vi "Update Occupied Area.vi"(8 "error in (no error)":errorcluster, 11 "UI Controller in":refnum<class "UI Controller.lvclass">) -> (0 "error out":errorcluster, 3 "UI Controller out":refnum<class "UI Controller.lvclass">)   [LabVIEW 2015, in "UI Controller.lvlib" / "UI Controller.lvclass"]
uses:
  UI Controller.lvclass
  UI Controller.lvclass/UI Controller.ctl
  <vilib>/ActorFrameworkMVC/View Controller/View Controller/View Controller.lvclass
panel:
  # "NOTICE -- YOU MUST LEAVE THIS NOTICE IN PLACE.\n\nCopyright (c) 2015, LIANG LIU Shawn.Liu.cn@gmail.com\nAll rights reserved.\n\nRedistribution and use in source and binary forms, with or without modification, are permitted provided that the following conditions are met:\n-Redistributions of source code must retain the above copyright notice, this list of conditions and the following disclaimer.\n-Redistributions in binary form must reproduce the above copyright notice, this list of conditions and the following disclaimer in the documentation and/or other materials provided with the distribution.\n-Neither the name of the eLp nor the names of its contributors may be used to endorse or promote products derived from this software without specific prior written permission.\n\nTHIS SOFTWARE IS PROVIDED BY THE COPYRIGHT HOLDERS AND CONTRIBUTORS \"AS IS\" AND ANY EXPRESS OR IMPLIED WARRANTIES, INCLUDING, BUT NOT LIMITED TO, THE IMPLIED WARRANTIES OF MERCHANTABILITY AND FITNESS FOR A PARTICULAR PURPOSE ARE DISCLAIMED. IN NO EVENT SHALL THE COPYRIGHT HOLDER OR CONTRIBUTORS BE LIABLE FOR ANY DIRECT, INDIRECT, INCIDENTAL, SPECIAL, EXEMPLARY, OR CONSEQUENTIAL DAMAGES (INCLUDING, BUT NOT LIMITED TO, PROCUREMENT OF SUBSTITUTE GOODS OR SERVICES; LOSS OF USE, DATA, OR PROFITS; OR BUSINESS INTERRUPTION) HOWEVER CAUSED AND ON ANY THEORY OF LIABILITY, WHETHER IN CONTRACT, STRICT LIABILITY, OR TORT (INCLUDING NEGLIGENCE OR OTHERWISE) ARISING IN ANY WAY OUT OF THE USE OF THIS SOFTWARE, EVEN IF ADVISED OF THE POSSIBILITY OF SUCH DAMAGE."
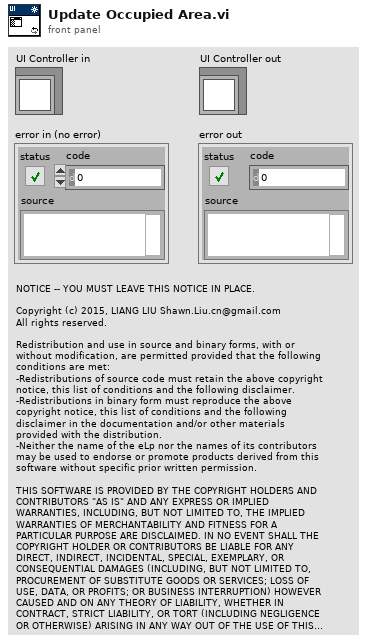
[diagram p1: front panel]
types:
  T1 = cluster{"left":i16, "top":i16, "right":i16, "bottom":i16}
  T2 = typedef "LVRectTypeDef.ctl" = cluster{"Left":i16, "Top":i16, "Right":i16, "Bottom":i16}
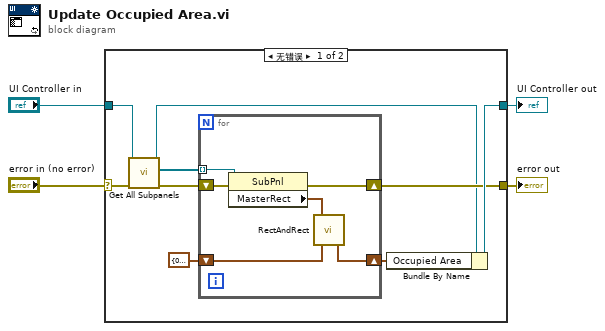
[diagram p0: block diagram]
diagram:
  n1 = case shown="无错误" "error in (no error)" {
    selector: "error in (no error)" -> [w6 w21]
    tunnel: [w11 w20] -> w4
    tunnel: [w10 w21] -> w3
    tunnel: "UI Controller in" -> [w5 w20]
    frame No Error {
      n2 = call <vilib>:"Get All Subpanels.vi"("error in (no error)"=w6, "View Controller in"=w5) -> ("error out"=w8:errorcluster, "Subpanels"=w7:refnum<vi>[], "View Controller out"=w9:refnum<class "UI Controller.lvclass">)  [unwired: 7 in]
      n3 = for {
        tunnel: w7 -> [w18] mode=indexing
        shift-right: [w17] -> w10
        shift-left: w8 -> [w19]
        shift-right: [w15] -> w12
        shift-left: T1 {"left"=0, "top"=0, "right"=0, "bottom"=0} ("union rect") -> [w16]
        n4 = property on="属性节点" class="SubPnl"(reference=w18, error in=w19) -> (error out=w17:errorcluster, "MasterRect"=w14:T2)  [unwired: 1 out]
        n5 = call <vilib>:"RectAndRect.vi"("rect b"=w16, "rect a"=w14) -> ("union rect"=w15:T1)
      }
      n6 = Bundle By Name(cluster=w9, "Occupied Area"=w12) -> (w11:refnum<class "UI Controller.lvclass">)
    }
    frame Error {
    }
  }
  "UI Controller out" <- w4
  "error out" <- w3
